vi "Resistor Calc Multi.vi"() -> ()   [LabVIEW 2010]
doc: "This VI will calculate the value of your resistor based on the colors of the bands on your resistor. Each tab will show the meaning of each band of your resistor. When you are finished, you will find the nominal value of the resistor, the tolerance value on your resistor, the change in resistance caused by temperature and the maximum and minimum values that your resistance can be. \n\n1.) Select your resistor style from the tabs above.\n2.) Select the specific colors that are on your resistor.\n3.) If you are using a 6 Band resistor, enter the operating temperature of the resistor to determine the additional resistance caused by the change in temperature.\n4.) Click \"Calculate\" to determine the resulting resistor values."
panel:
  in  "Stop":bool
  in  "Calculate":bool
  in  "Tab Control":T1(tab)
  in  "1st Digit":u16(ring)=1 items=["Black", "Brown", "Red", "Orange", "Yellow", "Green", "Blue", "Purple", "Grey", "White"]
  in  "2nd Digit":u16(ring)=1 items=["Black", "Brown", "Red", "Orange", "Yellow", "Green", "Blue", "Purple", "Grey", "White"]
  in  "Multiplier":dbl(ring)=10.0 items=["Silver"=0.01, "Gold"=0.1, "Black"=1.0, "Brown"=10.0, "Red"=100.0, "Orange"=1000.0, "Yellow"=10000.0, "Green"=100000.0, "Blue"=1000000.0, "Purple"=10000000.0]
  in  "Tolerance":dbl(ring)=0.01 items=["Silver"=0.1, "Gold"=0.05, "Brown"=0.01, "Red"=0.02, "Green"=0.005, "Blue"=0.0025, "Purple"=0.001]
  out "1":bool
  out "2":bool
  out "Mult":bool
  out "Tol":bool
  out "Mult 2":bool
  out "1 2":bool
  out "2 2":bool
  out "3 2":bool
  out "Tol 2":bool
  in  "1st Digit":u16(ring)=1 items=["Black", "Brown", "Red", "Orange", "Yellow", "Green", "Blue", "Purple", "Grey", "White"]
  in  "2nd Digit":u16(ring)=1 items=["Black", "Brown", "Red", "Orange", "Yellow", "Green", "Blue", "Purple", "Grey", "White"]
  in  "Multiplier":dbl(ring)=10.0 items=["Silver"=0.01, "Gold"=0.1, "Black"=1.0, "Brown"=10.0, "Red"=100.0, "Orange"=1000.0, "Yellow"=10000.0, "Green"=100000.0, "Blue"=1000000.0, "Purple"=10000000.0]
  in  "Tolerance":dbl(ring)=0.01 items=["Silver"=0.1, "Gold"=0.05, "Brown"=0.01, "Red"=0.02, "Green"=0.005, "Blue"=0.0025, "Purple"=0.001]
  in  "3rd Digit":u16(ring)=1 items=["Black", "Brown", "Red", "Orange", "Yellow", "Green", "Blue", "Purple", "Grey", "White"]
  in  "Temperature (C)":dbl=25.0
  out "Temp 3":bool
  out "Mult 3":bool
  out "1 3":bool
  out "23":bool
  out "33":bool
  out "Tol 3":bool
  in  "1st Digit":u16(ring)=1 items=["Black", "Brown", "Red", "Orange", "Yellow", "Green", "Blue", "Purple", "Grey", "White"]
  in  "2nd Digit":u16(ring)=1 items=["Black", "Brown", "Red", "Orange", "Yellow", "Green", "Blue", "Purple", "Grey", "White"]
  in  "Multiplier":dbl(ring)=10.0 items=["Silver"=0.01, "Gold"=0.1, "Black"=1.0, "Brown"=10.0, "Red"=100.0, "Orange"=1000.0, "Yellow"=10000.0, "Green"=100000.0, "Blue"=1000000.0, "Purple"=10000000.0]
  in  "Tolerance":dbl(ring)=0.01 items=["Silver"=0.1, "Gold"=0.05, "Brown"=0.01, "Red"=0.02, "Green"=0.005, "Blue"=0.0025, "Purple"=0.001]
  in  "3rd Digit":u16(ring)=1 items=["Black", "Brown", "Red", "Orange", "Yellow", "Green", "Blue", "Purple", "Grey", "White"]
  in  "Temp Coefficient":i32(ring)=100 items=["Brown"=100, "Red"=50, "Orange"=15, "Yellow"=25, "Blue"=10, "Purple"=5]
  out "Resistor Value":dbl=110.0 format="%#_6p"
  out "Tolerance Value":dbl=1.1 format="%#_6p"
  out "Lowest Actual Value":dbl=108.9 format="%#_6p"
  out "Highest Actual Value":dbl=111.1 format="%#_6p"
  out "Temp Adjustment":dbl format="%#_6p"
  # "This VI will calculate the value of your resistor based on the colors of the bands on your resistor. Each tab will show the meaning of each band of your resistor. When you are finished, you will find the nominal value of the resistor, the tolerance value on your resistor, the change in resistance caused by temperature and the maximum and minimum values that your resistance can be. \n\n1.) Select your resistor style from the tabs above.\n2.) Select the specific colors that are on your resistor.\n3.) If you are using a 6 Band resistor, enter the operating temperature of the resistor to determine the additional resistance caused by the change in temperature.\n4.) Click \"Calculate\" to determine the resulting resistor values."
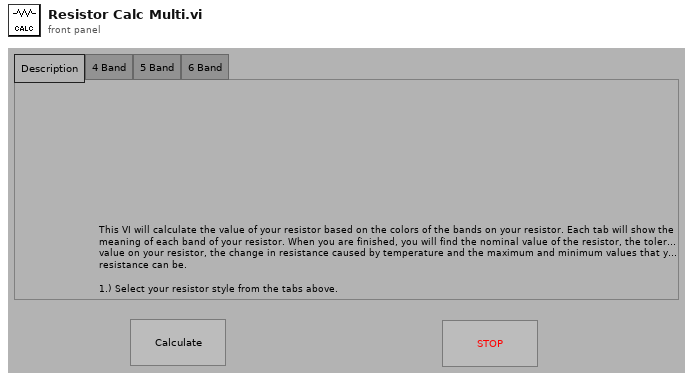
[diagram p1: front panel]
types:
  T1 = enum32{"Description", "4 Band", "5 Band", "6 Band", "Result"}
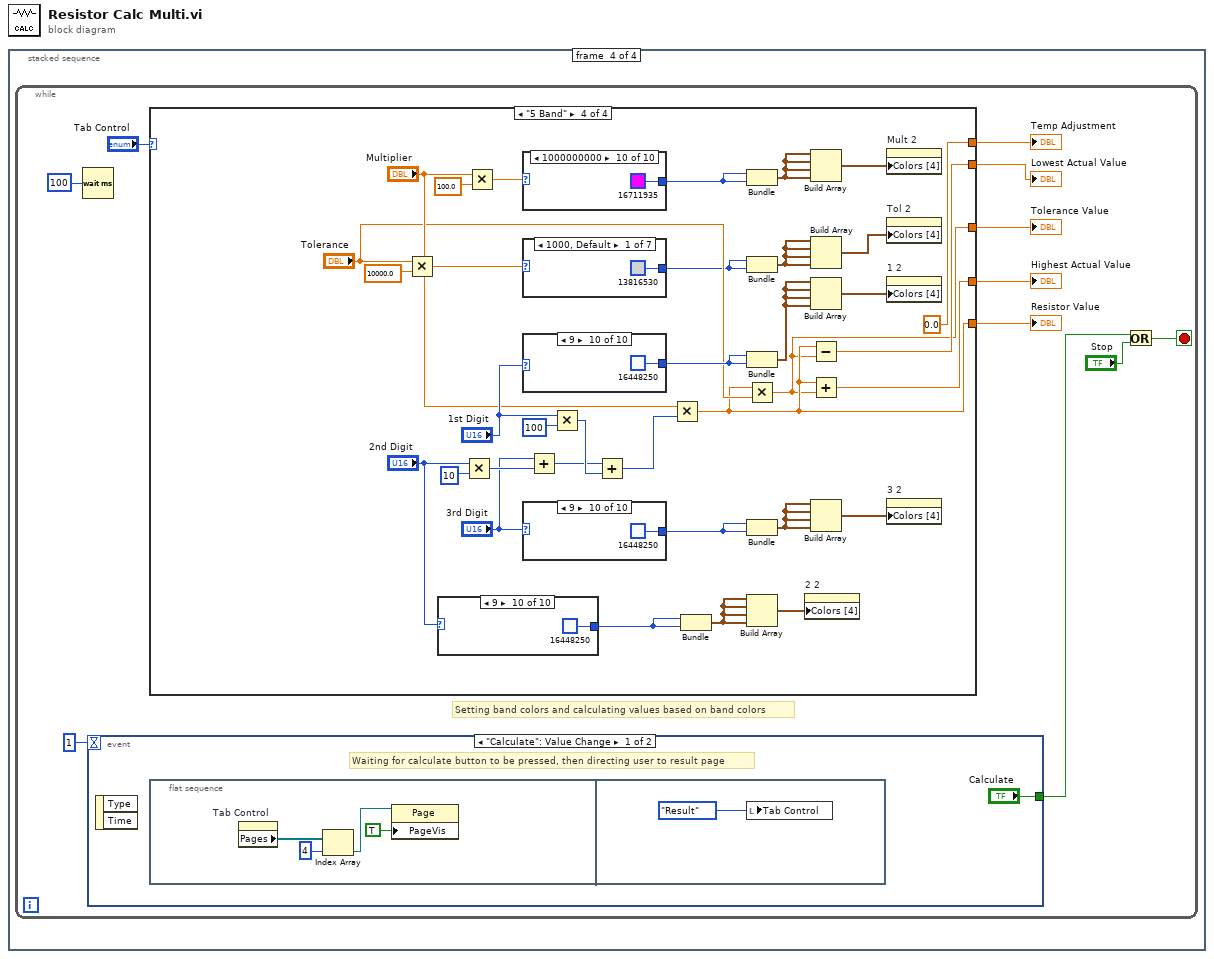
[diagram p0: block diagram]
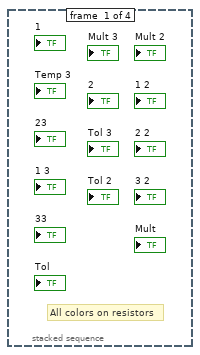
[diagram p2: hidden frame]
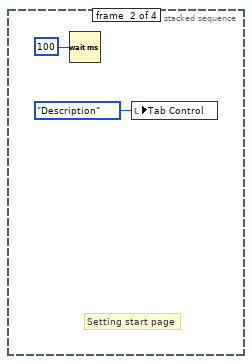
[diagram p3: hidden frame]
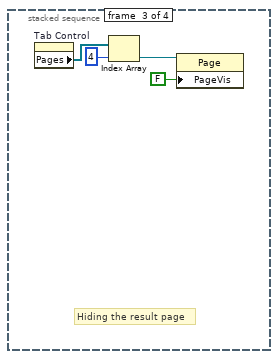
[diagram p4: hidden frame]
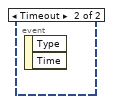
[diagram p5: hidden frame]
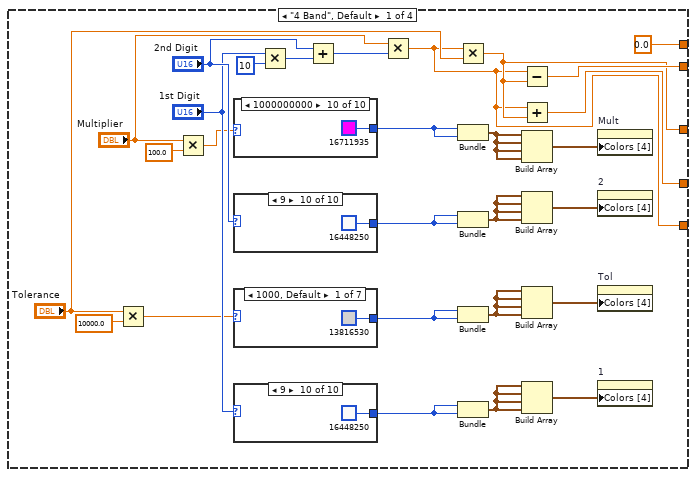
[diagram p6: hidden frame]
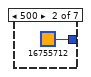
[diagram p7: hidden frame]
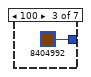
[diagram p8: hidden frame]
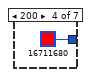
[diagram p9: hidden frame]
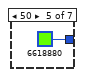
[diagram p10: hidden frame]
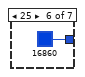
[diagram p11: hidden frame]
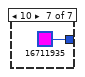
[diagram p12: hidden frame]
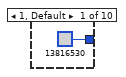
[diagram p13: hidden frame]
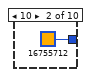
[diagram p14: hidden frame]
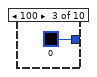
[diagram p15: hidden frame]
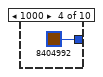
[diagram p16: hidden frame]
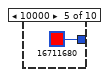
[diagram p17: hidden frame]
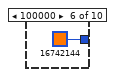
[diagram p18: hidden frame]
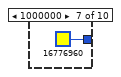
[diagram p19: hidden frame]
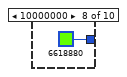
[diagram p20: hidden frame]
diagram:
  n1 = stacked-sequence {
    frame #0 {
      # "All colors on resistors"
    }
    frame #1 {
      # "Setting start page"
      n2 = Wait (ms)(milliseconds to wait=u32 100) -> ()  [unwired: 1 out]
      n3 = local write "Tab Control"(T1."Description" ("Tab Control")) -> ()
    }
    frame #2 {
      # "Hiding the result page"
      n4 = property on="Tab Control" class="TabCtl (strict)"() -> ("Pages"=w6:refnum<vi>[])  [unwired: 2 in, 2 out]
      n5 = Index Array(array=w6, index=4) -> (element=w5:refnum<vi>)
      n6 = property class="Page"(reference=w5, "PageVis"=FALSE ("Page Visible")) -> ()  [unwired: 1 in, 2 out]
    }
    frame #3 {
      n7 = while {
        stop <- w8 stop-if-true
        # "Setting band colors and calculating values based on band colors"
        n8 = Wait (ms)(milliseconds to wait=u32 100) -> ()  [unwired: 1 out]
        n9 = event shown="[0] \"Calculate\": Value Change" {
          selector: _ -> [_ _]
          dyn-events: _ -> [_ _]
          timeout: 1 -> [_ _]
          tunnel: ["Calculate" _] -> w16
          event "Calculate": Value Change {
            # "Waiting for calculate button to be pressed, then directing user to result page"
            n10 = event-data() -> ()  [unwired: 1 in, 2 out]
            n11 = flat-sequence {
              frame #0 {
                n12 = property on="Tab Control" class="TabCtl (strict)"() -> ("Pages"=w22:refnum<vi>[])  [unwired: 2 in, 2 out]
                n13 = Index Array(array=w22, index=4) -> (element=w21:refnum<vi>)
                n14 = property class="Page"(reference=w21, "PageVis"=TRUE ("Page Visible")) -> ()  [unwired: 1 in, 2 out]
              }
              frame #1 {
                n15 = local write "Tab Control"(T1."Result" ("Tab Control")) -> ()
              }
            }
          }
          event Timeout {
            n16 = event-data() -> ()  [unwired: 1 in, 2 out]
          }
        }
        n17 = case shown="\"5 Band\"" "Tab Control" {
          tunnel: [w28 w103 w186 w200] -> w15
          tunnel: [w27 w102 w186 w199] -> w14
          tunnel: [w26 w101 w186 w198] -> w13
          tunnel: [w25 w90 w186 w201] -> w12
          tunnel: [0.0 w91 w186 0.0] -> w11
          frame "4 Band", Default {
            n18 = Multiply(x="Tolerance", y=10000.0) -> (x*y=w34:dbl)
            n19 = Multiply(x="Multiplier", y=100.0) -> (x*y=w35:dbl)
            n20 = case shown="1000000000" w35 {
              tunnel: [u32 13816530 ("Color Box") u32 16755712 ("Color Box") u32 0 ("Color Box") u32 8404992 ("Color Box") u32 16711680 ("Color Box") u32 16742144 ("Color Box") u32 16776960 ("Color Box") u32 6618880 ("Color Box") u32 16860 ("Color Box") u32 16711935 ("Color Box")] -> w38
              frame 1, Default {
              }
              frame 10 {
              }
              frame 100 {
              }
              frame 1000 {
              }
              frame 10000 {
              }
              frame 100000 {
              }
              frame 1000000 {
              }
              frame 10000000 {
              }
              frame 100000000 {
              }
              frame 1000000000 {
              }
            }
            n21 = case shown="9" "2nd Digit" {
              tunnel: [u32 0 ("Color Box") u32 8404992 ("Color Box") u32 16711680 ("Color Box") u32 16742144 ("Color Box") u32 16776960 ("Color Box") u32 6618880 ("Color Box") u32 16860 ("Color Box") u32 16711935 ("Color Box") u32 12369084 ("Color Box") u32 16448250 ("Color Box")] -> w44
              frame 0, Default {
              }
              frame 1 {
              }
              frame 2 {
              }
              frame 3 {
              }
              frame 4 {
              }
              frame 5 {
              }
              frame 6 {
              }
              frame 7 {
              }
              frame 8 {
              }
              frame 9 {
              }
            }
            n22 = case shown="1000, Default" w34 {
              tunnel: [u32 13816530 ("Color Box") u32 16755712 ("Color Box") u32 8404992 ("Color Box") u32 16711680 ("Color Box") u32 6618880 ("Color Box") u32 16860 ("Color Box") u32 16711935 ("Color Box")] -> w30
              frame 1000, Default {
              }
              frame 500 {
              }
              frame 100 {
              }
              frame 200 {
              }
              frame 50 {
              }
              frame 25 {
              }
              frame 10 {
              }
            }
            n23 = case shown="9" "1st Digit" {
              tunnel: [u32 0 ("Color Box") u32 8404992 ("Color Box") u32 16711680 ("Color Box") u32 16742144 ("Color Box") u32 16776960 ("Color Box") u32 6618880 ("Color Box") u32 16860 ("Color Box") u32 16711935 ("Color Box") u32 12369084 ("Color Box") u32 16448250 ("Color Box")] -> w48
              frame 0, Default {
              }
              frame 1 {
              }
              frame 2 {
              }
              frame 3 {
              }
              frame 4 {
              }
              frame 5 {
              }
              frame 6 {
              }
              frame 7 {
              }
              frame 8 {
              }
              frame 9 {
              }
            }
            n24 = Multiply(x="1st Digit", y=10) -> (x*y=w50:i32)
            n25 = Add(x="2nd Digit", y=w50) -> (x+y=w49:i32)
            n26 = Multiply(x="Multiplier", y=w49) -> (x*y=w25:dbl)
            n27 = Multiply(x=w25, y="Tolerance") -> (x*y=w26:dbl)
            n28 = Bundle("Color Box"=w38, "Color Box"=w38) -> (w37:cluster{"Color Box":u32, "Color Box":u32})  [unwired: 1 in]
            n29 = Bundle("Color Box"=w44, "Color Box"=w44) -> (w45:cluster{"Color Box":u32, "Color Box":u32})  [unwired: 1 in]
            n30 = Bundle("Color Box"=w30, "Color Box"=w30) -> (w31:cluster{"Color Box":u32, "Color Box":u32})  [unwired: 1 in]
            n31 = Bundle("Color Box"=w48, "Color Box"=w48) -> (w47:cluster{"Color Box":u32, "Color Box":u32})  [unwired: 1 in]
            n32 = Subtract(x=w25, y=w26) -> (x-y=w27:dbl)
            n33 = Add(x=w25, y=w26) -> (x+y=w28:dbl)
            n34 = Build Array(w37, w37, w37, w37) -> (w36:cluster{"Color Box":u32, "Color Box":u32}[])
            n35 = Build Array(w45, w45, w45, w45) -> (w43:cluster{"Color Box":u32, "Color Box":u32}[])
            n36 = Build Array(w31, w31, w31, w31) -> (w29:cluster{"Color Box":u32, "Color Box":u32}[])
            n37 = Build Array(w47, w47, w47, w47) -> (w46:cluster{"Color Box":u32, "Color Box":u32}[])
            n38 = property on="Mult" class="Bool (strict)"("Colors [4]"=w36) -> ()  [unwired: 2 in, 2 out]
            n39 = property on="2" class="Bool (strict)"("Colors [4]"=w43) -> ()  [unwired: 2 in, 2 out]
            n40 = property on="Tol" class="Bool (strict)"("Colors [4]"=w29) -> ()  [unwired: 2 in, 2 out]
            n41 = property on="1" class="Bool (strict)"("Colors [4]"=w46) -> ()  [unwired: 2 in, 2 out]
          }
          frame "6 Band" {
            n42 = case shown="9" "2nd Digit" {
              tunnel: [u32 0 ("Color Box") u32 8404992 ("Color Box") u32 16711680 ("Color Box") u32 16742144 ("Color Box") u32 16776960 ("Color Box") u32 6618880 ("Color Box") u32 16860 ("Color Box") u32 16711935 ("Color Box") u32 12369084 ("Color Box") u32 16448250 ("Color Box")] -> w126
              frame 0, Default {
              }
              frame 1 {
              }
              frame 2 {
              }
              frame 3 {
              }
              frame 4 {
              }
              frame 5 {
              }
              frame 6 {
              }
              frame 7 {
              }
              frame 8 {
              }
              frame 9 {
              }
            }
            n43 = Multiply(x="2nd Digit", y=10) -> (x*y=w110:i32)
            n44 = case shown="9" "3rd Digit" {
              tunnel: [u32 0 ("Color Box") u32 8404992 ("Color Box") u32 16711680 ("Color Box") u32 16742144 ("Color Box") u32 16776960 ("Color Box") u32 6618880 ("Color Box") u32 16860 ("Color Box") u32 16711935 ("Color Box") u32 12369084 ("Color Box") u32 16448250 ("Color Box")] -> w111
              frame 0, Default {
              }
              frame 1 {
              }
              frame 2 {
              }
              frame 3 {
              }
              frame 4 {
              }
              frame 5 {
              }
              frame 6 {
              }
              frame 7 {
              }
              frame 8 {
              }
              frame 9 {
              }
            }
            n45 = case shown="9" "1st Digit" {
              tunnel: [u32 0 ("Color Box") u32 8404992 ("Color Box") u32 16711680 ("Color Box") u32 16742144 ("Color Box") u32 16776960 ("Color Box") u32 6618880 ("Color Box") u32 16860 ("Color Box") u32 16711935 ("Color Box") u32 12369084 ("Color Box") u32 16448250 ("Color Box")] -> w130
              frame 0, Default {
              }
              frame 1 {
              }
              frame 2 {
              }
              frame 3 {
              }
              frame 4 {
              }
              frame 5 {
              }
              frame 6 {
              }
              frame 7 {
              }
              frame 8 {
              }
              frame 9 {
              }
            }
            n46 = Add(x="3rd Digit", y=w110) -> (x+y=w107:i32)
            n47 = Multiply(x="1st Digit", y=100) -> (x*y=w131:i32)
            n48 = Add(x=w107, y=w131) -> (x+y=w92:i32)
            n49 = Multiply(x="Tolerance", y=10000.0) -> (x*y=w118:dbl)
            n50 = case shown="100, Default" "Temp Coefficient" {
              tunnel: [u32 8404992 ("Color Box") u32 16711680 ("Color Box") u32 16742144 ("Color Box") u32 16776960 ("Color Box") u32 16860 ("Color Box") u32 16711935 ("Color Box")] -> w99
              frame 100, Default {
              }
              frame 50 {
              }
              frame 15 {
              }
              frame 25 {
              }
              frame 10 {
              }
              frame 5 {
              }
            }
            n51 = Multiply(x="Temp Coefficient", y="Temperature (C)") -> (x*y=w94:dbl)
            n52 = Multiply(x="Multiplier", y=w92) -> (x*y=w90:dbl)
            n53 = Bundle("Color Box"=w126, "Color Box"=w126) -> (w127:cluster{"Color Box":u32, "Color Box":u32})  [unwired: 1 in]
            n54 = Multiply(x="Multiplier", y=100.0) -> (x*y=w119:dbl)
            n55 = case shown="1000000000" w119 {
              tunnel: [u32 13816530 ("Color Box") u32 16755712 ("Color Box") u32 0 ("Color Box") u32 8404992 ("Color Box") u32 16711680 ("Color Box") u32 16742144 ("Color Box") u32 16776960 ("Color Box") u32 6618880 ("Color Box") u32 16860 ("Color Box") u32 16711935 ("Color Box")] -> w121
              frame 1, Default {
              }
              frame 10 {
              }
              frame 100 {
              }
              frame 1000 {
              }
              frame 10000 {
              }
              frame 100000 {
              }
              frame 1000000 {
              }
              frame 10000000 {
              }
              frame 100000000 {
              }
              frame 1000000000 {
              }
            }
            n56 = case shown="1000, Default" w118 {
              tunnel: [u32 13816530 ("Color Box") u32 16755712 ("Color Box") u32 8404992 ("Color Box") u32 16711680 ("Color Box") u32 6618880 ("Color Box") u32 16860 ("Color Box") u32 16711935 ("Color Box")] -> w114
              frame 1000, Default {
              }
              frame 500 {
              }
              frame 100 {
              }
              frame 200 {
              }
              frame 50 {
              }
              frame 25 {
              }
              frame 10 {
              }
            }
            n57 = Multiply(x=w94, y=w90) -> (x*y=w93:dbl)
            n58 = Build Array(w127, w127, w127, w127) -> (w125:cluster{"Color Box":u32, "Color Box":u32}[])
            n59 = Bundle("Color Box"=w111, "Color Box"=w111) -> (w112:cluster{"Color Box":u32, "Color Box":u32})  [unwired: 1 in]
            n60 = Bundle("Color Box"=w130, "Color Box"=w130) -> (w129:cluster{"Color Box":u32, "Color Box":u32})  [unwired: 1 in]
            n61 = property on="23" class="Bool (strict)"("Colors [4]"=w125) -> ()  [unwired: 2 in, 2 out]
            n62 = Build Array(w112, w112, w112, w112) -> (w113:cluster{"Color Box":u32, "Color Box":u32}[])
            n63 = Build Array(w129, w129, w129, w129) -> (w128:cluster{"Color Box":u32, "Color Box":u32}[])
            n64 = property on="33" class="Bool (strict)"("Colors [4]"=w113) -> ()  [unwired: 2 in, 2 out]
            n65 = property on="1 3" class="Bool (strict)"("Colors [4]"=w128) -> ()  [unwired: 2 in, 2 out]
            n66 = Divide(x=w93, y=1000000.0) -> (x/y=w91:dbl)
            n67 = Bundle("Color Box"=w99, "Color Box"=w99) -> (w100:cluster{"Color Box":u32, "Color Box":u32})  [unwired: 1 in]
            n68 = Add(x=w91, y=w90) -> (x+y=w89:dbl)
            n69 = Build Array(w100, w100, w100, w100) -> (w98:cluster{"Color Box":u32, "Color Box":u32}[])
            n70 = Bundle("Color Box"=w121, "Color Box"=w121) -> (w120:cluster{"Color Box":u32, "Color Box":u32})  [unwired: 1 in]
            n71 = Multiply(x=w90, y="Tolerance") -> (x*y=w101:dbl)
            n72 = Bundle("Color Box"=w114, "Color Box"=w114) -> (w115:cluster{"Color Box":u32, "Color Box":u32})  [unwired: 1 in]
            n73 = property on="Temp 3" class="Bool (strict)"("Colors [4]"=w98) -> ()  [unwired: 2 in, 2 out]
            n74 = Build Array(w120, w120, w120, w120) -> (w105:cluster{"Color Box":u32, "Color Box":u32}[])
            n75 = Subtract(x=w89, y=w101) -> (x-y=w102:dbl)
            n76 = Add(x=w89, y=w101) -> (x+y=w103:dbl)
            n77 = Build Array(w115, w115, w115, w115) -> (w104:cluster{"Color Box":u32, "Color Box":u32}[])
            n78 = property on="Mult 3" class="Bool (strict)"("Colors [4]"=w105) -> ()  [unwired: 2 in, 2 out]
            n79 = property on="Tol 3" class="Bool (strict)"("Colors [4]"=w104) -> ()  [unwired: 2 in, 2 out]
          }
          frame "Result" {
            w186 = 0.0
          }
          frame "5 Band" {
            n80 = Multiply(x="Tolerance", y=10000.0) -> (x*y=w206:dbl)
            n81 = case shown="9" "2nd Digit" {
              tunnel: [u32 0 ("Color Box") u32 8404992 ("Color Box") u32 16711680 ("Color Box") u32 16742144 ("Color Box") u32 16776960 ("Color Box") u32 6618880 ("Color Box") u32 16860 ("Color Box") u32 16711935 ("Color Box") u32 12369084 ("Color Box") u32 16448250 ("Color Box")] -> w214
              frame 0, Default {
              }
              frame 1 {
              }
              frame 2 {
              }
              frame 3 {
              }
              frame 4 {
              }
              frame 5 {
              }
              frame 6 {
              }
              frame 7 {
              }
              frame 8 {
              }
              frame 9 {
              }
            }
            n82 = Multiply(x="2nd Digit", y=10) -> (x*y=w194:i32)
            n83 = Multiply(x="Multiplier", y=100.0) -> (x*y=w207:dbl)
            n84 = case shown="1000000000" w207 {
              tunnel: [u32 13816530 ("Color Box") u32 16755712 ("Color Box") u32 0 ("Color Box") u32 8404992 ("Color Box") u32 16711680 ("Color Box") u32 16742144 ("Color Box") u32 16776960 ("Color Box") u32 6618880 ("Color Box") u32 16860 ("Color Box") u32 16711935 ("Color Box")] -> w209
              frame 1, Default {
              }
              frame 10 {
              }
              frame 100 {
              }
              frame 1000 {
              }
              frame 10000 {
              }
              frame 100000 {
              }
              frame 1000000 {
              }
              frame 10000000 {
              }
              frame 100000000 {
              }
              frame 1000000000 {
              }
            }
            n85 = case shown="1000, Default" w206 {
              tunnel: [u32 13816530 ("Color Box") u32 16755712 ("Color Box") u32 8404992 ("Color Box") u32 16711680 ("Color Box") u32 6618880 ("Color Box") u32 16860 ("Color Box") u32 16711935 ("Color Box")] -> w202
              frame 1000, Default {
              }
              frame 500 {
              }
              frame 100 {
              }
              frame 200 {
              }
              frame 50 {
              }
              frame 25 {
              }
              frame 10 {
              }
            }
            n86 = case shown="9" "1st Digit" {
              tunnel: [u32 0 ("Color Box") u32 8404992 ("Color Box") u32 16711680 ("Color Box") u32 16742144 ("Color Box") u32 16776960 ("Color Box") u32 6618880 ("Color Box") u32 16860 ("Color Box") u32 16711935 ("Color Box") u32 12369084 ("Color Box") u32 16448250 ("Color Box")] -> w218
              frame 0, Default {
              }
              frame 1 {
              }
              frame 2 {
              }
              frame 3 {
              }
              frame 4 {
              }
              frame 5 {
              }
              frame 6 {
              }
              frame 7 {
              }
              frame 8 {
              }
              frame 9 {
              }
            }
            n87 = case shown="9" "3rd Digit" {
              tunnel: [u32 0 ("Color Box") u32 8404992 ("Color Box") u32 16711680 ("Color Box") u32 16742144 ("Color Box") u32 16776960 ("Color Box") u32 6618880 ("Color Box") u32 16860 ("Color Box") u32 16711935 ("Color Box") u32 12369084 ("Color Box") u32 16448250 ("Color Box")] -> w195
              frame 0, Default {
              }
              frame 1 {
              }
              frame 2 {
              }
              frame 3 {
              }
              frame 4 {
              }
              frame 5 {
              }
              frame 6 {
              }
              frame 7 {
              }
              frame 8 {
              }
              frame 9 {
              }
            }
            n88 = Add(x="3rd Digit", y=w194) -> (x+y=w191:i32)
            n89 = Multiply(x="1st Digit", y=100) -> (x*y=w220:i32)
            n90 = Add(x=w191, y=w220) -> (x+y=w219:i32)
            n91 = Multiply(x="Multiplier", y=w219) -> (x*y=w201:dbl)
            n92 = Bundle("Color Box"=w214, "Color Box"=w214) -> (w215:cluster{"Color Box":u32, "Color Box":u32})  [unwired: 1 in]
            n93 = Bundle("Color Box"=w209, "Color Box"=w209) -> (w208:cluster{"Color Box":u32, "Color Box":u32})  [unwired: 1 in]
            n94 = Bundle("Color Box"=w202, "Color Box"=w202) -> (w203:cluster{"Color Box":u32, "Color Box":u32})  [unwired: 1 in]
            n95 = Bundle("Color Box"=w218, "Color Box"=w218) -> (w217:cluster{"Color Box":u32, "Color Box":u32})  [unwired: 1 in]
            n96 = Multiply(x=w201, y="Tolerance") -> (x*y=w198:dbl)
            n97 = Bundle("Color Box"=w195, "Color Box"=w195) -> (w196:cluster{"Color Box":u32, "Color Box":u32})  [unwired: 1 in]
            n98 = Build Array(w215, w215, w215, w215) -> (w213:cluster{"Color Box":u32, "Color Box":u32}[])
            n99 = property on="2 2" class="Bool (strict)"("Colors [4]"=w213) -> ()  [unwired: 2 in, 2 out]
            n100 = Build Array(w208, w208, w208, w208) -> (w189:cluster{"Color Box":u32, "Color Box":u32}[])
            n101 = Build Array(w203, w203, w203, w203) -> (w188:cluster{"Color Box":u32, "Color Box":u32}[])
            n102 = Build Array(w217, w217, w217, w217) -> (w216:cluster{"Color Box":u32, "Color Box":u32}[])
            n103 = Subtract(x=w201, y=w198) -> (x-y=w199:dbl)
            n104 = Add(x=w201, y=w198) -> (x+y=w200:dbl)
            n105 = Build Array(w196, w196, w196, w196) -> (w197:cluster{"Color Box":u32, "Color Box":u32}[])
            n106 = property on="Mult 2" class="Bool (strict)"("Colors [4]"=w189) -> ()  [unwired: 2 in, 2 out]
            n107 = property on="Tol 2" class="Bool (strict)"("Colors [4]"=w188) -> ()  [unwired: 2 in, 2 out]
            n108 = property on="1 2" class="Bool (strict)"("Colors [4]"=w216) -> ()  [unwired: 2 in, 2 out]
            n109 = property on="3 2" class="Bool (strict)"("Colors [4]"=w197) -> ()  [unwired: 2 in, 2 out]
          }
        }
        "Highest Actual Value" <- w15
        "Lowest Actual Value" <- w14
        "Tolerance Value" <- w13
        "Resistor Value" <- w12
        "Temp Adjustment" <- w11
        n110 = Or(x=w16, y="Stop") -> (x .or. y?=w8:bool)
      }
    }
  }
